vi "ReadDataCluster.vi"(8 "error in (no error)":errorcluster) -> (0 "error out":errorcluster, 2 "DataCluster":cluster{"CounterNum":i32})   [LabVIEW 2013, in "Data.lvclass"]
uses:
  Data.lvclass
  Singleton.lvclass/Singleton.lvclass/Singleton.ctl
  Data.lvclass/Data.ctl
  Singleton.lvclass/Constructor.vi
  Singleton.lvclass/Singleton.lvclass
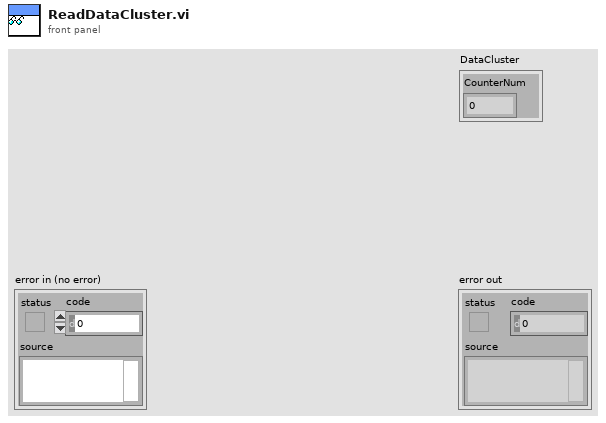
[diagram p1: front panel]
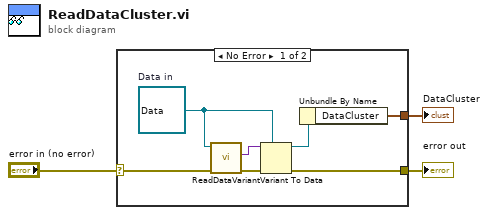
[diagram p0: block diagram]
diagram:
  n1 = case shown="No Error" "error in (no error)" {
    selector: "error in (no error)" -> [w5 w11]
    tunnel: [w6 w11] -> w2
    tunnel: [w10 _] -> w1
    frame No Error {
      w4 = refnum<class "Data.lvclass"> refnum  # Data in
      n2 = call "ReadDataVariant.vi"("error in (no error)"=w5, "Singleton.lvclass In"=w4) -> ("error out"=w9:errorcluster, "DataVariant"=w8:variant)  [unwired: 7 in, 1 out]
      n3 = Variant To Data(error in=w9, type=w4, Variant=w8) -> (data=w7:refnum<class "Data.lvclass">, error out=w6:errorcluster)
      n4 = Unbundle By Name(w7) -> ("DataCluster"=w10:cluster{"CounterNum":i32})
    }
    frame Error {
    }
  }
  "error out" <- w2
  "DataCluster" <- w1
